vi "onLock.vi"(8 "error in (no error)":errorcluster, 11 "ReadyState in":refnum<class "ReadyState.lvclass">) -> (0 "error out":errorcluster, 2 "String":string, 3 "ReadyState out":refnum<class "ReadyState.lvclass">)   [LabVIEW 2016, in "ReadyState.lvclass"]
uses:
  ReadyState.lvclass
  State Class/State.lvclass
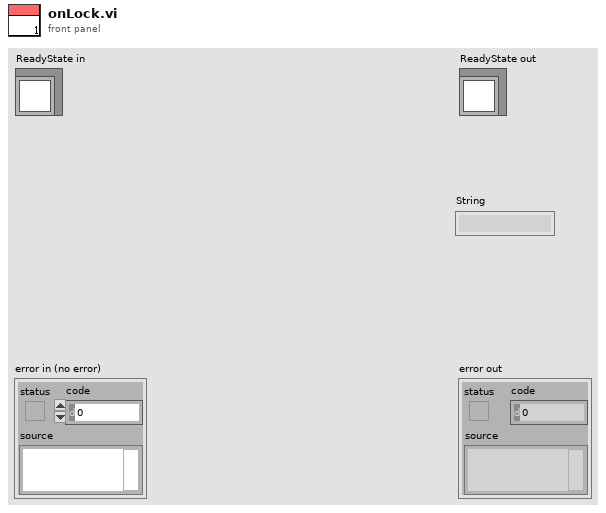
[diagram p1: front panel]
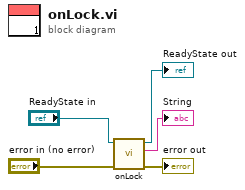
[diagram p0: block diagram]
diagram:
  n1 = call-parent "onLock.vi"("error in (no error)"="error in (no error)", "State in"="ReadyState in") -> ("error out"=→"error out":errorcluster, "String"=→"String":string, "State out"=→"ReadyState out":refnum<class "ReadyState.lvclass">)  [unwired: 7 in]
